vi "NEW数据采集传输系统.vi"() -> ()   [LabVIEW 2016, in "数据传输系统-05.lvlib"]
uses:
  <vilib>/Utility/miscctls.llb/LVPointTypeDef.ctl
  <vilib>/Utility/error.llb/whitespace.ctl
  <vilib>/picture/picture.llb/imagedata.ctl
  <vilib>/Utility/config.llb/NI_LVConfig.lvlib
  update/update.lvlib
panel:
  out "剖面数据补发":bool
  out "日志信息补发":bool
  out "数据补发":bool
  in  "自动更新":bool
  in  "数据补传":bool caption="确定"
  out "数据库打开失败次数":dbl
  out "与工控通信指示灯":bool
  in  "判断数据反馈":enum16{"非严格判断", "严格判断", "不判断"}(ring)
  in  "暂停上传":bool
  in  "配置表":bool caption="确定"
  in  "updateconfiguration":T1={"主机"="27.154.58.30", "用户"="update", "密码"="std23506", "远程路径"="数据传输系统\\平台数据传输系统.exe", "下载文件名"="平台数据传输系统.exe", "软件版本"=""}
  out "标题显示":string
  in  "更新":bool
  in  "系统编码选择框":string(combo)="地表水质量监测"
  in  "数据发送通道":enum16{"TCP", "VISA"}(ring)
  in  "baud rate":u32=9600 caption="波特率"
  in  "VISA resource name":refnum<visa-resource-name> caption="VISA资源名称"
  in  "实时数据发送时间间隔/min":i32=1
  in  "数据组合发送":bool
  in  "2011发送":bool
  in  "数据发送协议":enum16{"2005-212协议", "2017-212协议"}(ring)=enum."2017-212协议"
  in  "重发时间":T2(ring)
  in  "重发日期":T3(ring)
  in  "开机启动":bool
  in  "每周自动重发":bool=TRUE
  in  "确定":bool
  in  "返回":bool
  in  "PW":string
  in  "MN":string
  in  "PORT":string
  in  "IP":string
  in  "站点设备":string
  in  "站点名称":string
  out "设置超时时间/min":i32=1
  out "状态信息":T4={"1st Error to Convert "=63, "步骤 "=enum."发送数据", "元素"="实时数据", "TCP服务端掉线计数"=0, "TCP掉线时间节点"="2019/05/08 15:24:17"} {"1st Error to Convert" items=["无错误", "参数错误", "内存已满", "超出区域", "文件结束", "文件已打开", "一般文件IO错误", "未找到文件", "文件权限错误", "磁盘已满", "路径副本", "打开过多文件", "未启用", "未找到资源文件", "无法添加资源", "未找到资源", "未找到图像", "图像内存错误", "画笔不存在", "配置错误类型", "配置未找到解析段", "配置解析错误", "配置内存错误", "错误外部代码格式", "错误外部代码偏移量", "外部代码不存在", "空窗口", "销毁窗口错误", "空菜单", "打印已中止", "错误打印记录", "打印驱动程序错误", "打印时窗口错误", "打印时内存错误", "打印对话框错误", "一般打印错误", "无效设备引用句柄", "设备未找到", "设备参数错误", "设备单位错误", "无法打开设备", "设备调用已中止", "一般错误", "用户已取消", "对象ID过低", "对象ID过高", "对象不在堆中", "未知的堆", "错误DefProc ID", "DefProc不在表格中", "范围外信息", "空方法", "未知信息", "不支持管理器调用", "错误地址", "连接过程中", "连接超时", "连接过程中", "不支持网络属性", "网络错误", "正在使用的地址", "系统缺少内存", "连接已中止", "连接已拒绝", "连接未建立", "连接已建立", "连接已关闭", "初始化错误（交互应用程序管理器）", "错误事件发生", "等待无约束事件发生处理程序", "事件发生队列溢出", "错误路径", "未发出信号量", "未识别类型（交互应用程序管理器）"]}
  out "数据接收超时指示灯":bool
  out "空闲时间/s":string
  out "系统时间":string
  out "实时小时数据上传":bool
  out "系统状态改变":bool
  out "软件版本":string
  out "掉线指示":bool
  out "核查数据上传":bool
  out "配置信息":T5
  in  "参数配置":bool
  out "反控数据发送":bool
  out "读取报文显示":string
  out "发送报文显示":string
  out "心跳包":bool
  out "通信状态":bool
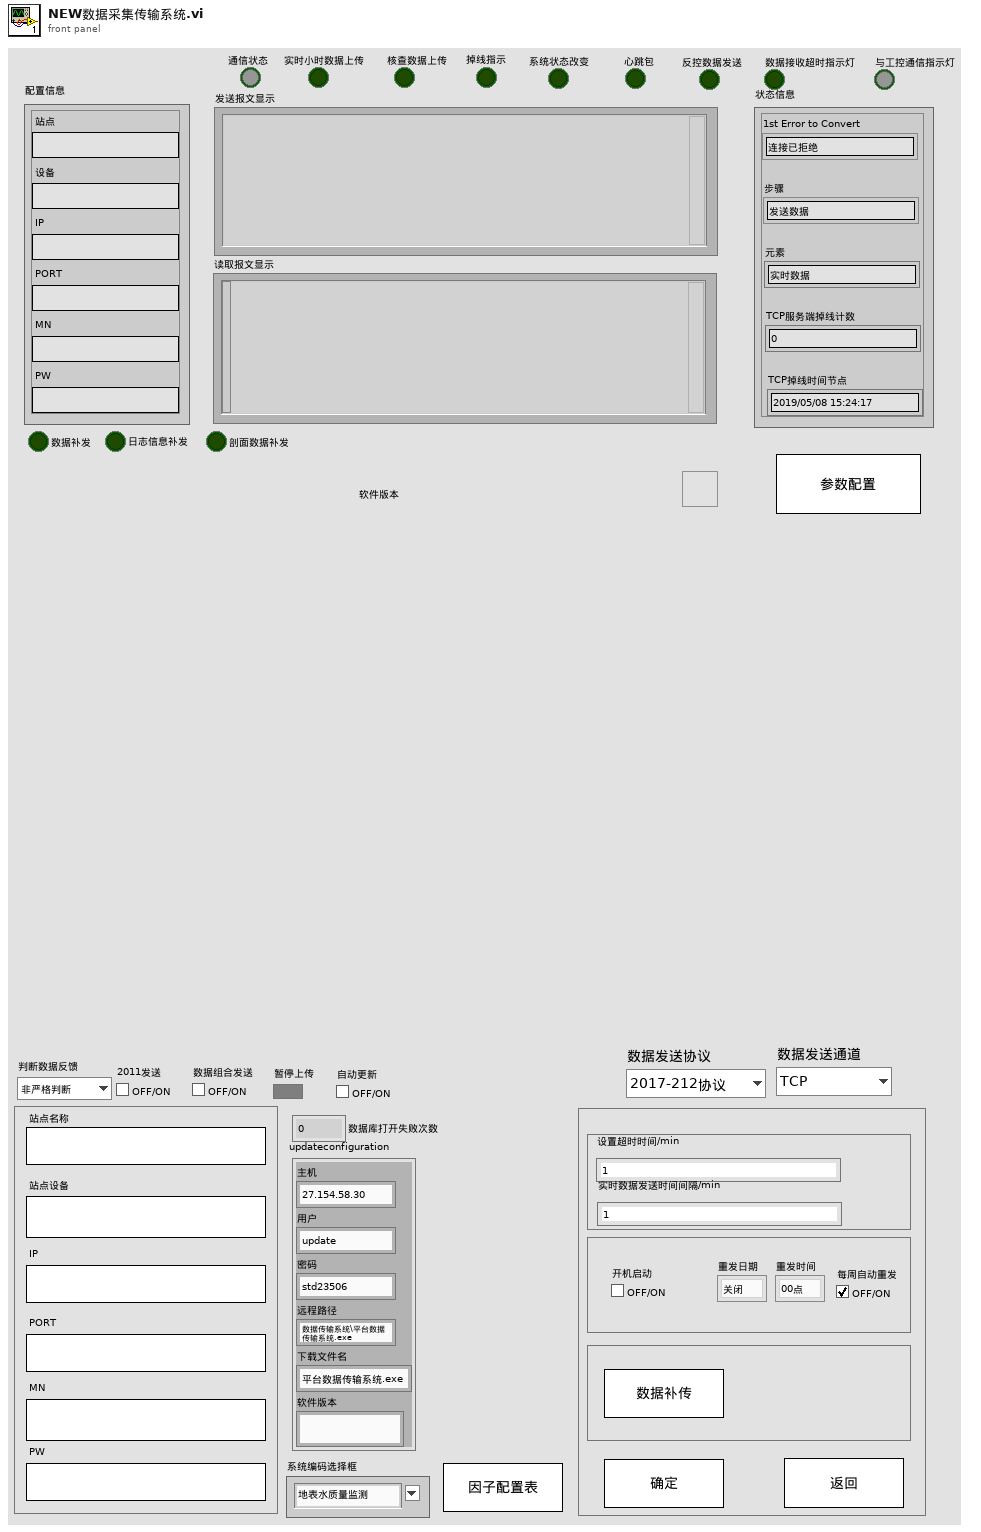
[diagram p1: front panel]
types:
  T1 = cluster{"主机":string, "用户":string, "密码":string, "远程路径":string, "下载文件名":string, "软件版本":string}
  T2 = enum16{"00点", "01点", "02点", "03点", "04点", "05点", "06点", "07点", "08点", "09点", "10点", "11点", "12点", "13点", "14点", "15点", "16点", "17点", "18点", "19点", "20点", "21点", "22点", "23点"}
  T3 = enum16{"关闭", "星期日", "星期一", "星期二", "星期三", "星期四", "星期五", "星期六"}
  T4 = cluster{"1st Error to Convert ":i32, "步骤 ":enum16{"打开连接", "发送数据", "读取数据", "数据处理", "关闭连接"}, "元素":string, "TCP服务端掉线计数":i32, "TCP掉线时间节点":string}
  T5 = cluster{"站点":string, "设备":string, "IP":string, "PORT":string, "MN":string, "PW":string}
  T6 = typedef "imagedata.ctl" = cluster{"image type":i32, "image depth":i32, "image":u8[], "mask":u8[], "colors":u32[], "Rectangle":cluster{"left":i16, "top":i16, "right":i16, "bottom":i16}}
  T7 = typedef "LVPointTypeDef.ctl" = cluster{"Horizontal":i16, "Vertical":i16}
  T8 = cluster{"setini":string, "sysini":string, "hechaini":string, "actualwrite":string, "actualread":string, "datasent":string, "反控命令信息队列":string, "反控与仪器交互":string}
  T9 = cluster{"配置表格[0]":string, "配置表格[1]":string, "配置表格[2]":string, "配置表格[3]":string, "配置表格[4]":string, "配置表格[5]":string, "配置表格[6]":string, "配置表格[7]":string, "配置表格[8]":string, "配置表格[9]":string, "配置表格[10]":string, "配置表格[11]":string, "配置表格[12]":string, "配置表格[13]":string, "配置表格[14]":string, "配置表格[15]":string, "配置表格[16]":string, "配置表格[17]":string, "配置表格[18]":string, "配置表格[19]":string, "配置表格[20]":string, "配置表格[21]":string, "配置表格[22]":string, "配置表格[23]":string, "配置表格[24]":string, "配置表格[25]":string, "配置表格[26]":string, "配置表格[27]":string, "配置表格[28]":string, "配置表格[29]":string, "配置表格[30]":string, "配置表格[31]":string, "配置表格[32]":string, "配置表格[33]":string, "配置表格[34]":string}
  T10 = cluster{"[0]":dbl, "[1]":dbl, "[2]":dbl, "[3]":dbl, "[4]":dbl, "[5]":dbl, "[6]":dbl, "[7]":dbl, "[8]":dbl, "[9]":dbl, "[10]":dbl, "[11]":dbl, "[12]":dbl, "[13]":dbl, "[14]":dbl, "[15]":dbl, "[16]":dbl, "[17]":dbl, "[18]":dbl, "[19]":dbl, "[20]":dbl, "[21]":dbl, "[22]":dbl, "[23]":dbl, "[24]":dbl, "[25]":dbl, "[26]":dbl, "[27]":dbl, "[28]":dbl, "[29]":dbl, "[30]":dbl, "[31]":dbl, "[32]":dbl, "[33]":dbl, "[34]":dbl}
  T11 = cluster{"时间标识":timestamp, "设备":string, "日志信息":string, "流程参数":string}
  T12 = cluster{"host":string, "port":u16, "user":string, "password":string, "远端地址":string}
  T13 = typedef "NI_LVConfig.lvlib/Config Data RefNum.ctl" = refnum<k1>
  T14 = cluster{"[0]":string, "[1]":string, "[2]":string, "[3]":string, "[4]":string, "[5]":string, "[6]":string}
  T15 = cluster{"[0]":string, "[1]":string, "[2]":string, "[3]":string, "[4]":string, "[5]":string, "[6]":string, "[7]":string, "[8]":string}
  T16 = cluster{"[0]":string, "[1]":string, "[2]":string, "[3]":string, "[4]":string, "[5]":string}
  T17 = cluster{"[0]":string, "[1]":string, "[2]":string, "[3]":string, "[4]":string, "[5]":string, "[6]":string, "[7]":string, "[8]":string, "[9]":string, "[10]":string, "[11]":string, "[12]":string, "[13]":string, "[14]":string, "[15]":string}
  T18 = cluster{"[0]":string, "[1]":string, "[2]":string, "[3]":string, "[4]":string, "[5]":string, "[6]":string, "[7]":string, "[8]":string, "[9]":string, "[10]":string, "[11]":string, "[12]":string, "[13]":string}
  T19 = cluster{"[0]":string, "[1]":string, "[2]":string, "[3]":string, "[4]":string, "[5]":string, "[6]":string, "[7]":string, "[8]":string, "[9]":string, "[10]":string, "[11]":string, "[12]":string, "[13]":string, "[14]":string, "[15]":string, "[16]":string, "[17]":string, "[18]":string, "[19]":string, "[20]":string, "[21]":string, "[22]":string, "[23]":string, "[24]":string, "[25]":string, "[26]":string, "[27]":string, "[28]":string, "[29]":string, "[30]":string, "[31]":string, "[32]":string, "[33]":string, "[34]":string}
  T20 = typedef "whitespace.ctl" = u16
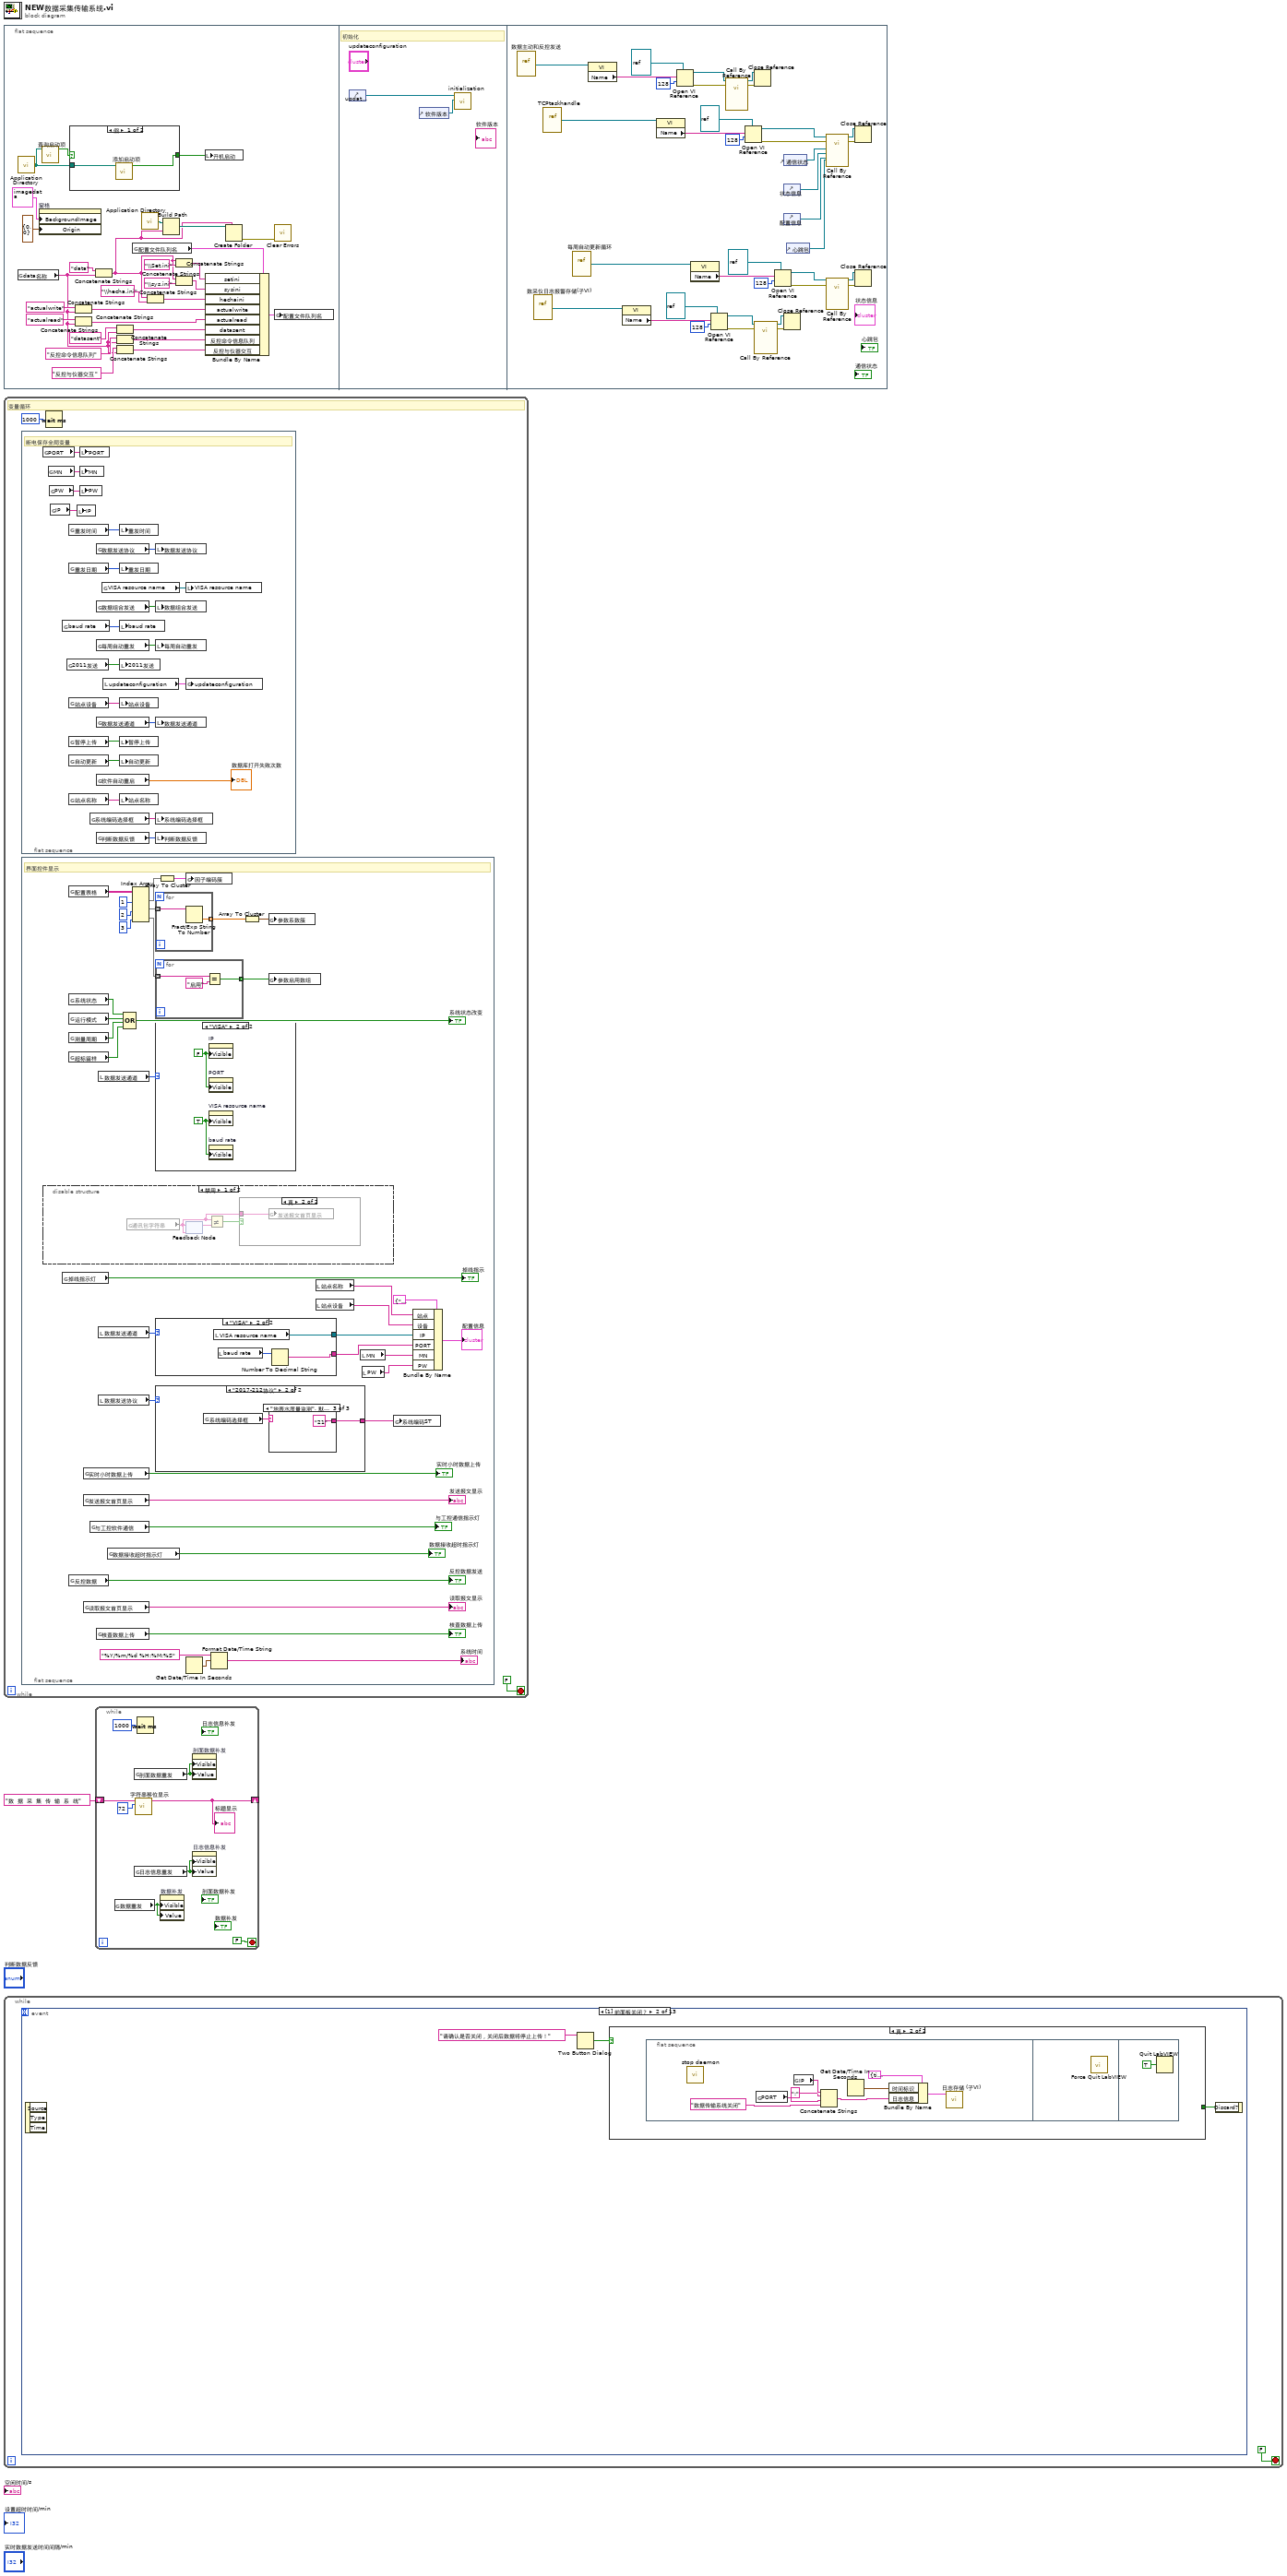
[diagram p0: block diagram]
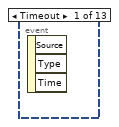
[diagram p2: hidden frame]
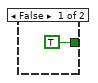
[diagram p3: hidden frame]
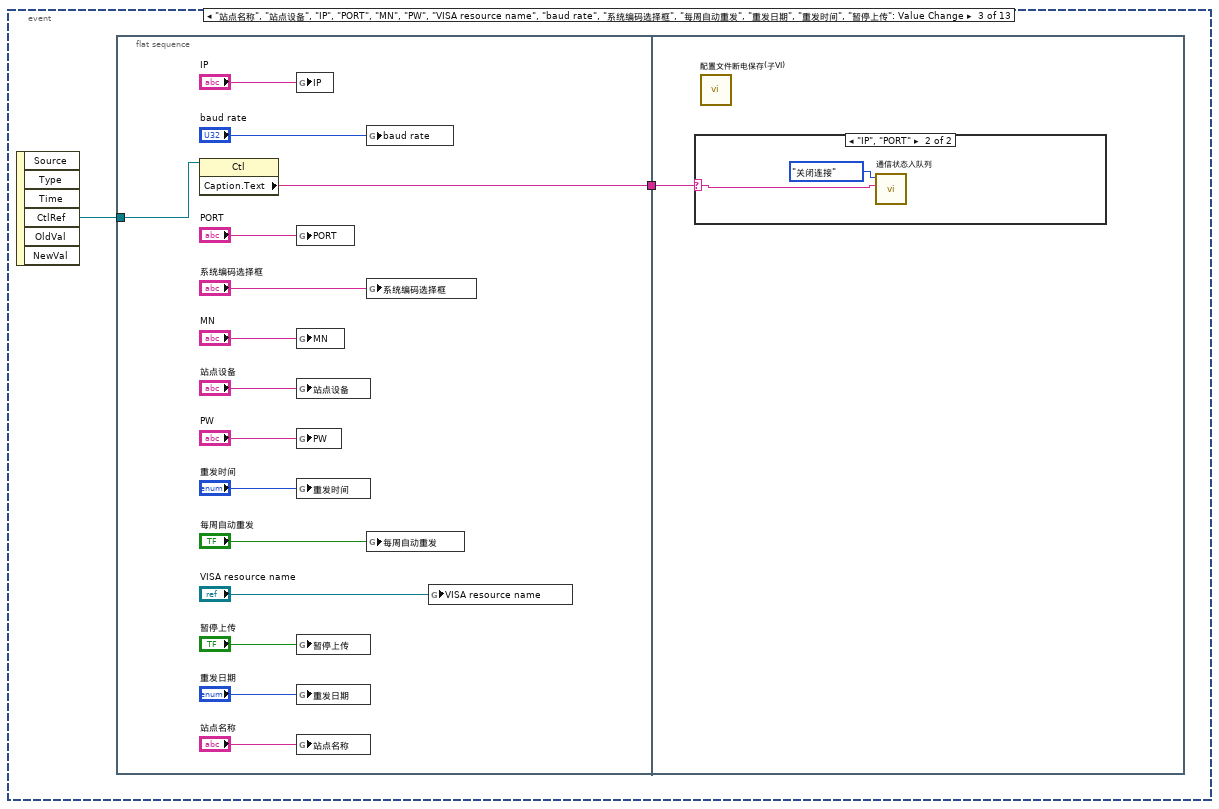
[diagram p4: hidden frame]
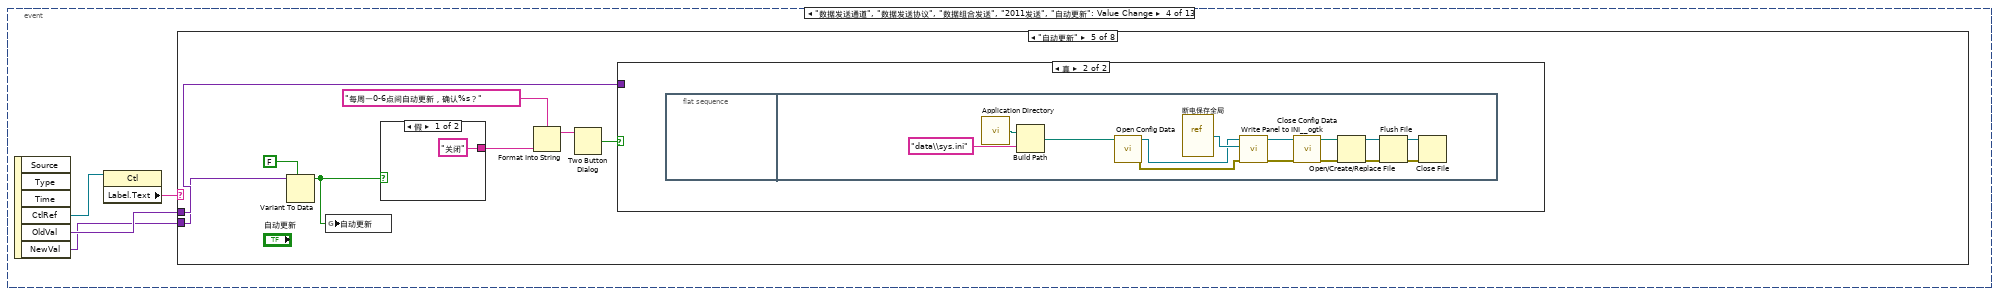
[diagram p6: hidden frame]
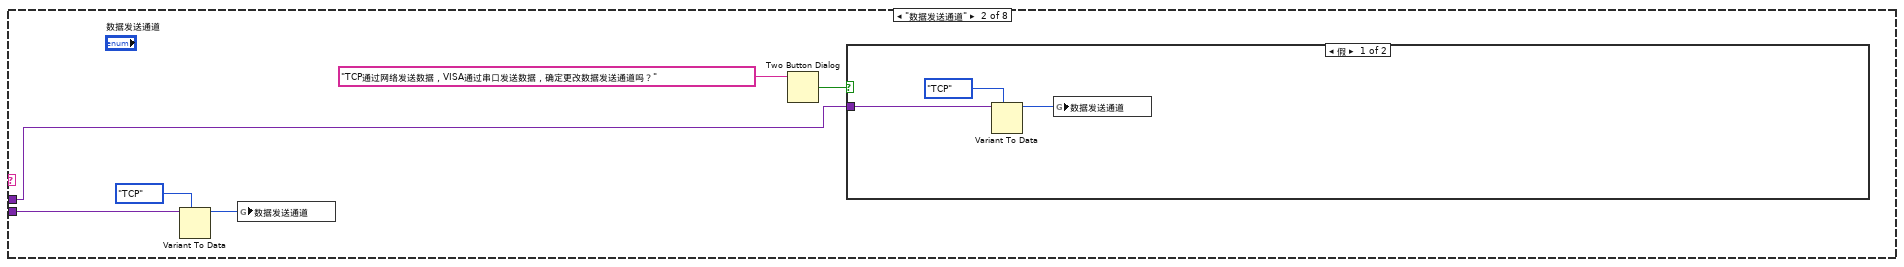
[diagram p8: hidden frame]
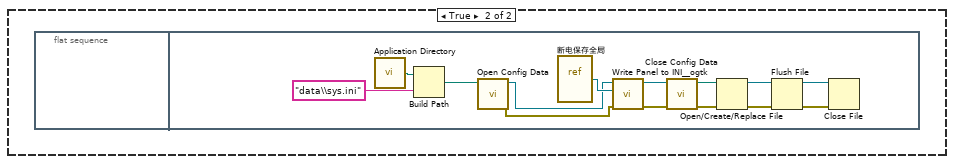
[diagram p9: hidden frame]
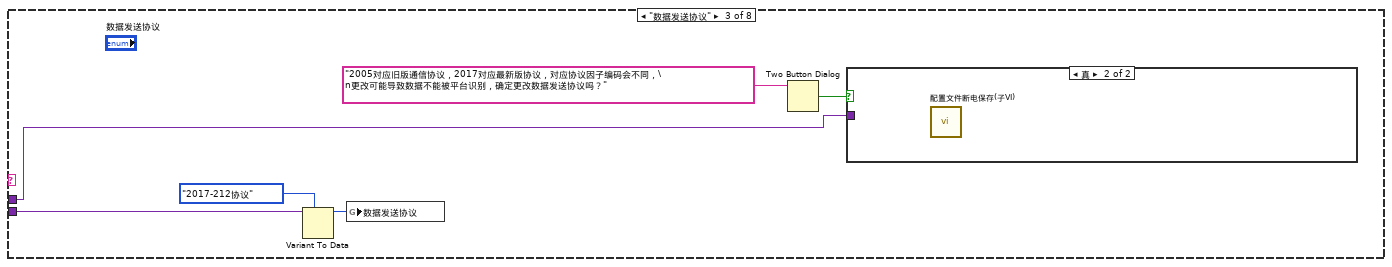
[diagram p10: hidden frame]
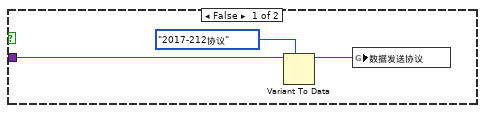
[diagram p11: hidden frame]
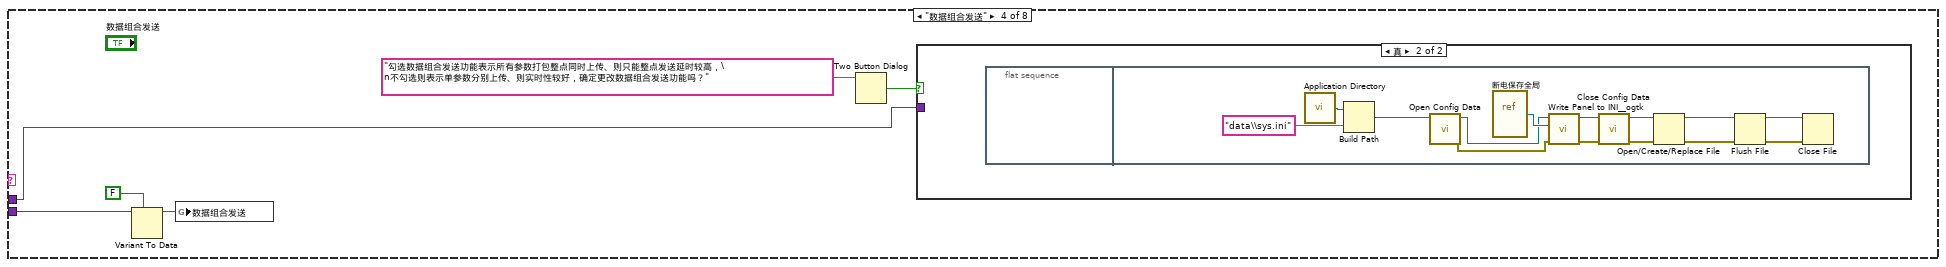
[diagram p12: hidden frame]
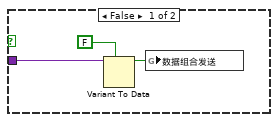
[diagram p13: hidden frame]
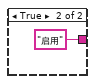
[diagram p14: hidden frame]
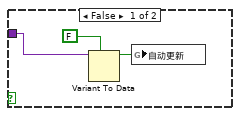
[diagram p15: hidden frame]
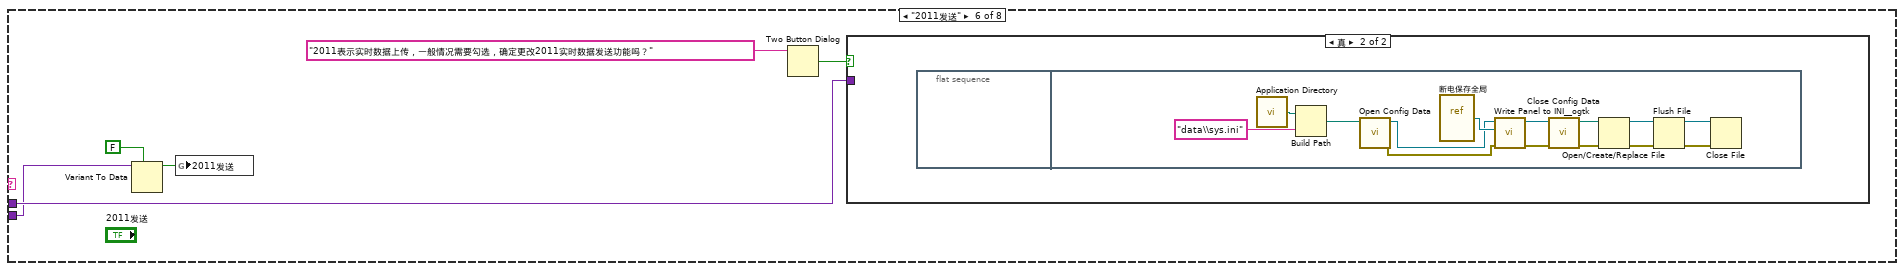
[diagram p16: hidden frame]
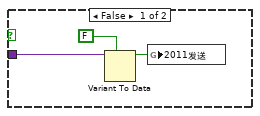
[diagram p17: hidden frame]
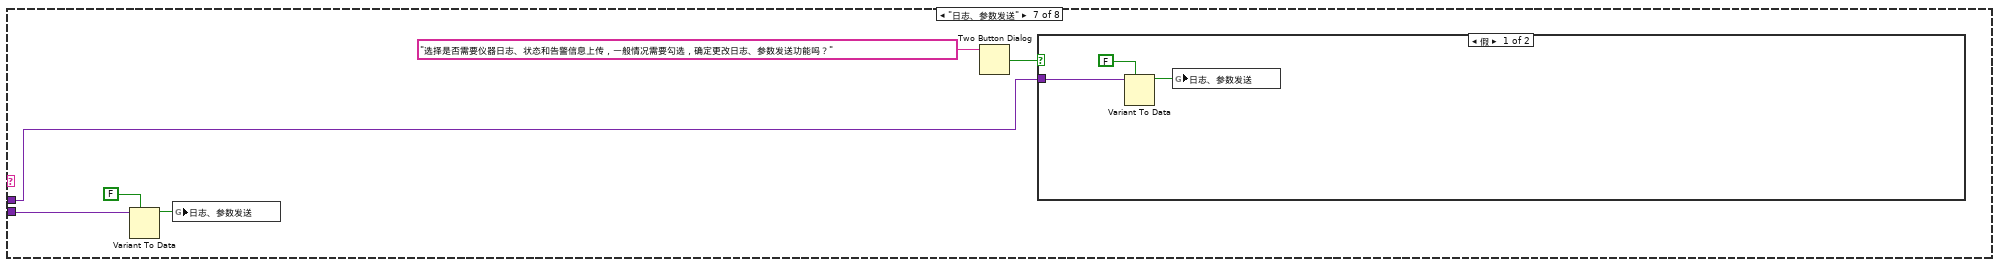
[diagram p18: hidden frame]
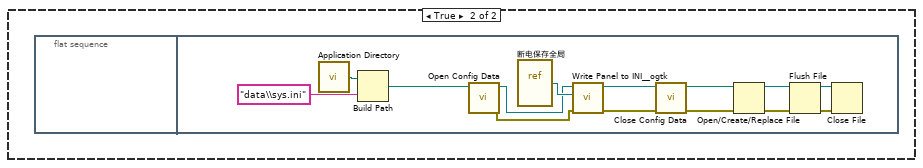
[diagram p19: hidden frame]
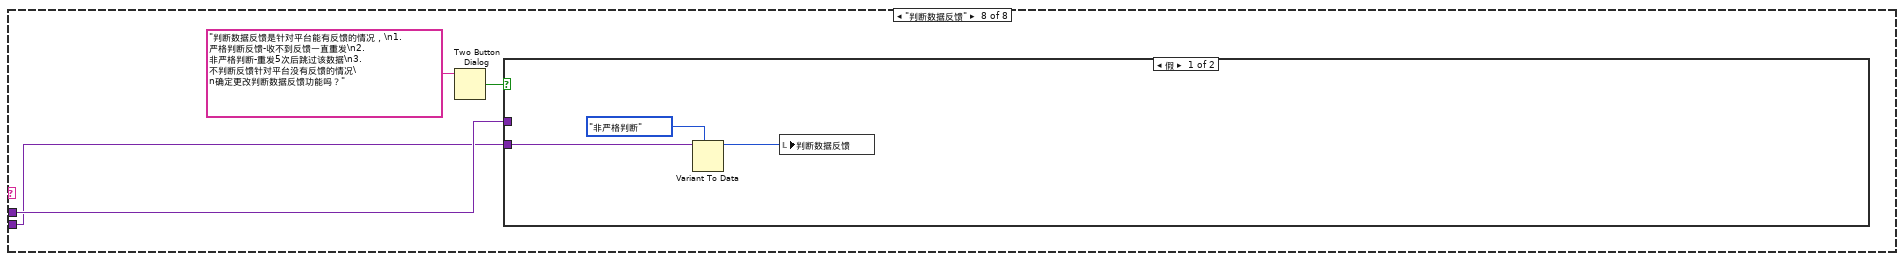
[diagram p20: hidden frame]
diagram:
  n1 = flat-sequence {
    frame #0 {
      n2 = global read "断电保存全局.vi" "data名称"() -> (w2:string)
      n3 = call <vilib>:"Application Directory.vi"() -> ("Application Directory"=w6:path)
      n4 = property on="窗格" class="Pane"("BackgroundImage"=T6 {"image type"=0, "image depth"=24, "image"=array[12288000 elements], "mask"=[], "colors"=[], "Rectangle"={"left"=0, "top"=0, "right"=2560, "bottom"=1600}} ("image data"), "Origin"=T7 {"Horizontal"=0, "Vertical"=0} ("原点")) -> ()  [unwired: 2 in, 2 out]
      n5 = call "查询启动项.vi"("启动文件路径"=w6) -> ("包含启动项"=w5:bool)  [unwired: 9 in, 1 out]
      n6 = case shown="假" w5 {
        selector: w5 -> [_ w33]
        tunnel: w6 -> [w32 _]
        tunnel: [w31 w33] -> w4
        frame False {
          n7 = call "添加启动项.vi"("启动文件路径"=w32) -> ("添加成功标记"=w31:bool)  [unwired: 9 in, 1 out]
        }
        frame True {
        }
      }
      n8 = Concatenate Strings("actualwrite" ("名称（未命名）"), w2) -> (w18:string)
      n9 = Concatenate Strings("actualread" ("名称（未命名）"), w2) -> (w16:string)
      n10 = Concatenate Strings("data" ("对话框窗口（创建文件夹）"), w2) -> (w23:string)
      n11 = Concatenate Strings("datasent" ("名称（未命名）"), w2) -> (w14:string)
      n12 = Concatenate Strings("反控命令信息队列" ("名称（未命名）"), w2) -> (w8:string)
      n13 = Concatenate Strings("反控与仪器交互" ("名称（未命名）"), w2) -> (w9:string)
      n14 = global read "断电保存全局.vi" "配置文件队列名"() -> (w13:T8)
      n15 = call <vilib>:"Application Directory.vi"() -> ("Application Directory"=w29:path)
      n16 = Concatenate Strings(w23, "\\hecha.ini" ("名称或相对路径")) -> (w21:string)
      n17 = Build Path(base path=w29, name or relative path=w23) -> (appended path=w28:path)
      n18 = Concatenate Strings(w23, "\\Set.ini" ("名称或相对路径")) -> (w25:string)
      n19 = Concatenate Strings(w23, "\\sys.ini" ("名称或相对路径")) -> (w22:string)
      n20 = local write "开机启动"(w4) -> ()
      n21 = Bundle By Name(cluster=w13, "setini"=w25, "sysini"=w22, "hechaini"=w21, "actualwrite"=w18, "actualread"=w16, "datasent"=w14, "反控命令信息队列"=w8, "反控与仪器交互"=w9) -> (w12:T8)
      n22 = Create Folder(prompt (Create Folder)=w23, path (use dialog)=w28) -> (error out=w27:errorcluster)  [unwired: 1 in, 2 out]
      n23 = call <vilib>:"Clear Errors.vi"("error in (no error)"=w27) -> ()  [unwired: 5 in, 2 out]
      n24 = global write "断电保存全局.vi" "配置文件队列名"(w12) -> ()
    }
    frame #1 {
      # "初始化"
      n25 = control-ref of="updateconfiguration"() -> (w35:refnum<vi>)
      n26 = control-ref of="软件版本"() -> (w34:refnum<vi>)
      n27 = call "initialization.vi"("软件版本"=w34, "updateconfiguration"=w35) -> ()  [unwired: 9 in]
    }
    frame #2 {
      n28 = vi-ref "数据主动和反控发送.vi"() -> (w63:refnum<vi>)
      n29 = vi-ref "数采仪日志报警存储(子VI).vi"() -> (w64:refnum<vi>)
      n30 = vi-ref "TCPtaskhandle.vi"() -> (w40:refnum<vi>)
      n31 = vi-ref "每周自动更新循环.vi"() -> (w55:refnum<vi>)
      n32 = property class="VI"(reference=w63) -> ("Name"=w62:string)  [unwired: 1 in, 2 out]
      n33 = property class="VI"(reference=w64) -> ("Name"=w71:string)  [unwired: 1 in, 2 out]
      n34 = property class="VI"(reference=w40) -> ("Name"=w47:string)  [unwired: 1 in, 2 out]
      n35 = Open VI Reference(type specifier VI Refnum (for type only)=refnum<vi> refnum, vi path=w62, options=128 ("选项")) -> (vi reference=w60:refnum<vi>, error out=w58:errorcluster)  [unwired: 3 in]
      n36 = property class="VI"(reference=w55) -> ("Name"=w48:string)  [unwired: 1 in, 2 out]
      n37 = Open VI Reference(type specifier VI Refnum (for type only)=refnum<vi> refnum, vi path=w71, options=128 ("选项")) -> (vi reference=w69:refnum<vi>, error out=w67:errorcluster)  [unwired: 3 in]
      n38 = call-by-ref "?"(reference=w60, error in=w58) -> (reference out=w56:refnum<vi>, error out=w57:errorcluster)  [unwired: 12 in]
      n39 = Open VI Reference(type specifier VI Refnum (for type only)=refnum<vi> refnum, vi path=w47, options=128 ("选项")) -> (vi reference=w45:refnum<vi>, error out=w43:errorcluster)  [unwired: 3 in]
      n40 = Close Reference(reference=w56, error in (no error)=w57) -> ()  [unwired: 1 out]
      n41 = call-by-ref "?"(reference=w69, error in=w67) -> (reference out=w65:refnum<vi>, error out=w66:errorcluster)  [unwired: 12 in]
      n42 = Open VI Reference(type specifier VI Refnum (for type only)=refnum<vi> refnum, vi path=w48, options=128 ("选项")) -> (vi reference=w50:refnum<vi>, error out=w52:errorcluster)  [unwired: 3 in]
      n43 = control-ref of="通信状态"() -> (w39:refnum<vi>)
      n44 = control-ref of="状态信息"() -> (w38:refnum<vi>)
      n45 = control-ref of="配置信息"() -> (w37:refnum<vi>)
      n46 = Close Reference(reference=w65, error in (no error)=w66) -> ()  [unwired: 1 out]
      n47 = control-ref of="心跳包"() -> (w36:refnum<vi>)
      n48 = call-by-ref "?"(reference=w45, error in=w43, "心跳包"=w36, "配置信息"=w37, "状态信息"=w38, "通信状态"=w39) -> (reference out=w41:refnum<vi>, error out=w42:errorcluster)  [unwired: 8 in]
      n49 = call-by-ref "?"(reference=w50, error in=w52) -> (reference out=w54:refnum<vi>, error out=w53:errorcluster)  [unwired: 12 in]
      n50 = Close Reference(reference=w41, error in (no error)=w42) -> ()  [unwired: 1 out]
      n51 = Close Reference(reference=w54, error in (no error)=w53) -> ()  [unwired: 1 out]
    }
  }
  n52 = while {
    stop <- FALSE stop-if-true
    # "变量循环"
    n53 = flat-sequence {
      frame #0 {
        # "断电保存全局变量"
        n54 = global read "断电保存全局.vi" "PORT"() -> (w158:string)
        n55 = global read "断电保存全局.vi" "MN"() -> (w157:string)
        n56 = global read "断电保存全局.vi" "PW"() -> (w156:string)
        n57 = global read "断电保存全局.vi" "IP"() -> (w159:string)
        n58 = global read "断电保存全局.vi" "baud rate"() -> (w154:u32)
        n59 = global read "断电保存全局.vi" "2011发送"() -> (w150:bool)
        n60 = global read "断电保存全局.vi" "重发时间"() -> (w145:T2)
        n61 = global read "断电保存全局.vi" "重发日期"() -> (w152:T3)
        n62 = global read "断电保存全局.vi" "站点设备"() -> (w160:string)
        n63 = global read "断电保存全局.vi" "暂停上传"() -> (w143:bool)
        n64 = global read "断电保存全局.vi" "自动更新"() -> (w141:bool)
        n65 = global read "断电保存全局.vi" "站点名称"() -> (w161:string)
        n66 = local write "IP"(w159) -> ()
        n67 = local write "PORT"(w158) -> ()
        n68 = local write "MN"(w157) -> ()
        n69 = local write "PW"(w156) -> ()
        n70 = global read "断电保存全局.vi" "系统编码选择框"() -> (w146:string)
        n71 = global read "断电保存全局.vi" "数据发送协议"() -> (w148:enum16{"2005-212协议", "2017-212协议"})
        n72 = global read "断电保存全局.vi" "数据组合发送"() -> (w149:bool)
        n73 = global read "断电保存全局.vi" "每周自动重发"() -> (w153:bool)
        n74 = global read "断电保存全局.vi" "数据发送通道"() -> (w147:enum16{"TCP", "VISA"})
        n75 = global read "全局1.vi" "软件自动重启"() -> (→"数据库打开失败次数":dbl)
        n76 = global read "断电保存全局.vi" "判断数据反馈"() -> (w151:enum16{"非严格判断", "严格判断", "不判断"})
        n77 = global read "断电保存全局.vi" "VISA resource name"() -> (w155:refnum<visa-resource-name>)
        n78 = local read "updateconfiguration"() -> (w144:T1)
        n79 = local write "重发时间"(w145) -> ()
        n80 = local write "重发日期"(w152) -> ()
        n81 = local write "baud rate"(w154) -> ()
        n82 = local write "2011发送"(w150) -> ()
        n83 = local write "站点设备"(w160) -> ()
        n84 = local write "暂停上传"(w143) -> ()
        n85 = local write "自动更新"(w141) -> ()
        n86 = local write "站点名称"(w161) -> ()
        n87 = local write "数据发送协议"(w148) -> ()
        n88 = local write "数据组合发送"(w149) -> ()
        n89 = local write "每周自动重发"(w153) -> ()
        n90 = local write "数据发送通道"(w147) -> ()
        n91 = local write "系统编码选择框"(w146) -> ()
        n92 = local write "判断数据反馈"(w151) -> ()
        n93 = local write "VISA resource name"(w155) -> ()
        n94 = global write "更新全局变量.vi" "updateconfiguration"(w144) -> ()
      }
    }
    n95 = flat-sequence {
      frame #0 {
        # "界面控件显示"
        n96 = disable-structure shown="禁用" {
          frame Disabled {
            n97 = global read "全局1.vi" "通讯包字符串"() -> (w114:string)
            n98 = feedback #1(w114) -> (w115:string)
            n99 = feedback-in #1(w114) -> ()
            n100 = Not Equal?(x=w114, y=w115) -> (x != y?=w113:bool)
            n101 = case shown="真" w113 {
              tunnel: w114 -> [_ w116]
              frame False {
              }
              frame True {
                n102 = global write "全局1.vi" "发送报文首页显示"(w116) -> ()
              }
            }
          }
          frame Enabled {
          }
        }
        n103 = global read "全局 数据发送重叠.vi" "掉线指示灯"() -> (→"掉线指示":bool)
        n104 = global read "断电保存全局.vi" "配置表格"() -> (w84:string[][])
        n105 = global read "全局1.vi" "系统状态"() -> (w86:bool)
        n106 = global read "全局1.vi" "运行模式"() -> (w87:bool)
        n107 = global read "全局1.vi" "测量周期"() -> (w88:bool)
        n108 = global read "全局1.vi" "超标留样"() -> (w89:bool)
        n109 = global read "全局1.vi" "反控数据"() -> (→"反控数据发送":bool)
        n110 = global read "全局1.vi" "实时小时数据上传"() -> (→"实时小时数据上传":bool)
        n111 = global read "全局1.vi" "发送报文首页显示"() -> (→"发送报文显示":string)
        n112 = global read "全局1.vi" "读取报文首页显示"() -> (→"读取报文显示":string)
        n113 = global read "全局1.vi" "与工控软件通信"() -> (→"与工控通信指示灯":bool)
        n114 = global read "全局1.vi" "核查数据上传"() -> (→"核查数据上传":bool)
        n115 = local read "数据发送通道"() -> (w94:enum16{"TCP", "VISA"})
        n116 = local read "数据发送通道"() -> (w112:enum16{"TCP", "VISA"})
        n117 = local read "数据发送协议"() -> (w101:enum16{"2005-212协议", "2017-212协议"})
        n118 = global read "全局 数据发送重叠.vi" "数据接收超时指示灯"() -> (→"数据接收超时指示灯":bool)
        n119 = Compound Arithmetic op=OR ("复合运算")(w86, w87, w88, w89) -> (→"系统状态改变":bool)
        n120 = Index Array(array=w84, index (col) #1=1 ("禁用的索引 (列)"), index (col) #2=2 ("索引 (列)"), index (col) #3=3 ("索引 (列)")) -> (element #1=w82:string[], element #2=w76:string[], element #3=w78:string[])  [unwired: 3 in]
        n121 = for {
          tunnel: w76 -> [w118] mode=indexing
          tunnel: [w117] -> w75 mode=indexing
          n122 = Fract/Exp String To Number(string=w118) -> (number=w117:dbl)  [unwired: 3 in, 1 out]
        }
        n123 = for {
          tunnel: w78 -> [w121] mode=indexing
          tunnel: [w119] -> w77 mode=indexing
          n124 = Equal?(x=w121, y="启用") -> (x = y?=w119:bool)
        }
        n125 = case shown="\"VISA\"" w94 {
          frame "TCP", Default {
            w122 = TRUE ("可见")
            w123 = FALSE ("可见")
            n126 = property on="IP" class="Str"("Visible"=w122) -> ()  [unwired: 2 in, 2 out]
            n127 = property on="PORT" class="Str"("Visible"=w122) -> ()  [unwired: 2 in, 2 out]
            n128 = property on="VISA resource name" class="VISAName"("Visible"=w123) -> ()  [unwired: 2 in, 2 out]
            n129 = property on="baud rate" class="DigNum (严格)"("Visible"=w123) -> ()  [unwired: 2 in, 2 out]
          }
          frame "VISA" {
            w124 = FALSE ("可见")
            w125 = TRUE ("可见")
            n130 = property on="IP" class="Str"("Visible"=w124) -> ()  [unwired: 2 in, 2 out]
            n131 = property on="PORT" class="Str"("Visible"=w124) -> ()  [unwired: 2 in, 2 out]
            n132 = property on="VISA resource name" class="VISAName"("Visible"=w125) -> ()  [unwired: 2 in, 2 out]
            n133 = property on="baud rate" class="DigNum (严格)"("Visible"=w125) -> ()  [unwired: 2 in, 2 out]
          }
        }
        n134 = case shown="\"VISA\"" w112 {
          tunnel: [w137 w140] -> w109
          tunnel: [w136 w138] -> w106
          frame "TCP", Default {
            n135 = local read "PORT"() -> (w136:string)
            n136 = local read "IP"() -> (w137:string)
          }
          frame "VISA" {
            n137 = local read "VISA resource name"() -> (w140:refnum<visa-resource-name>)
            n138 = local read "baud rate"() -> (w139:u32)
            n139 = Number To Decimal String(number=w139) -> (decimal integer string=w138:string)  [unwired: 1 in]
          }
        }
        n140 = case shown="\"2017-212协议\"" w101 {
          tunnel: [w126 w131] -> w100
          frame "2005-212协议", Default {
            n141 = global read "断电保存全局.vi" "系统编码选择框"() -> (w127:string)
            n142 = case shown="\"地表水体污染源\"" w127 {
              tunnel: ["52" ("设备编码MN") "32" ("设备编码MN") "21" ("设备编码MN")] -> w126
              frame "污水排放过程监测" {
              }
              frame "地表水体污染源" {
              }
              frame "地表水质量监测", Default {
              }
            }
          }
          frame "2017-212协议" {
            n143 = global read "断电保存全局.vi" "系统编码选择框"() -> (w132:string)
            n144 = case shown="\"地表水质量监测\", 默认" w132 {
              tunnel: ["52" ("设备编码MN") "32" ("设备编码MN") "21" ("设备编码MN")] -> w131
              frame "污水排放过程监测" {
              }
              frame "地表水体污染源" {
              }
              frame "地表水质量监测", Default {
              }
            }
          }
        }
        n145 = Array To Cluster(array=w82) -> (cluster=w85:T9)
        n146 = global write "断电保存全局.vi" "因子编码簇"(w85) -> ()
        n147 = Get Date/Time In Seconds() -> (seconds since 1Jan1904=w102:timestamp)
        n148 = Format Date/Time String(time format string (%c)="%Y/%m/%d %H:%M:%S" ("时间格式字符串(%c)"), seconds (now)=w102) -> (date/time string=→"系统时间":string)  [unwired: 1 in]
        n149 = Array To Cluster(array=w75) -> (cluster=w79:T10)
        n150 = global write "断电保存全局.vi" "参数系数簇"(w79) -> ()
        n151 = global write "断电保存全局.vi" "参数启用数组"(w77) -> ()
        n152 = local read "站点名称"() -> (w108:string)
        n153 = local read "站点设备"() -> (w107:string)
        n154 = local read "MN"() -> (w105:string)
        n155 = local read "PW"() -> (w104:string)
        n156 = global write "全局1.vi" "系统编码ST"(w100) -> ()
        n157 = Bundle By Name(cluster=T5 {"站点"="", "设备"="", "IP"="", "PORT"="", "MN"="", "PW"=""} ("配置信息"), "站点"=w108, "设备"=w107, "IP"=w109, "PORT"=w106, "MN"=w105, "PW"=w104) -> (→"配置信息":T5)
      }
    }
    n158 = Wait (ms)(milliseconds to wait=u32 1000 ("等待时间（毫秒）")) -> ()  [unwired: 1 out]
  }
  n159 = while {
    stop <- FALSE stop-if-true
    n160 = event shown="[1] 前面板关闭？" {
      selector: _ -> [_ _ _ _ _ _ _ _ _ _ _ _ _]
      dyn-events: _ -> [_ _ _ _ _ _ _ _ _ _ _ _ _]
      timeout: _ -> [_ _ _ _ _ _ _ _ _ _ _ _ _]
      event Timeout {
        n161 = event-data() -> ()  [unwired: 1 in, 3 out]
      }
      event Panel Close? {
        n162 = event-data() -> ()  [unwired: 1 in, 3 out]
        n163 = Two Button Dialog(message="请确认是否关闭，关闭后数据将停止上传！" ("消息")) -> (T button?=w164:bool)  [unwired: 2 in]
        n164 = case shown="真" w164 {
          tunnel: [TRUE _] -> w163
          frame False {
          }
          frame True {
            n165 = flat-sequence {
              frame #0 {
                n166 = call "stop daemon.vi"() -> ()  [unwired: 11 in, 1 out]
                n167 = global read "断电保存全局.vi" "PORT"() -> (w170:string)
                n168 = global read "断电保存全局.vi" "IP"() -> (w172:string)
                n169 = Concatenate Strings(w172, ":", w170, "数据传输系统关闭" ("日志信息")) -> (w168:string)
                n170 = Get Date/Time In Seconds() -> (seconds since 1Jan1904=w174:timestamp)
                n171 = Bundle By Name(cluster=T11 {"时间标识"=timestamp(0 s since 1904-01-01), "设备"="数采仪", "日志信息"="", "流程参数"=""} ("data in"), "时间标识"=w174, "日志信息"=w168) -> (w173:T11)
                n172 = call "日志存储 (子VI).vi"("data in"=w173) -> ()  [unwired: 11 in]
              }
              frame #1 {
                n173 = call "Force Quit LabVIEW.vi"() -> ()  [unwired: 10 in, 2 out]
              }
              frame #2 {
                n174 = Quit LabVIEW(quit? (T)=TRUE ("退出？(T)")) -> ()
              }
            }
          }
        }
        n175 = event-data("Discard?"=w163) -> ()  [unwired: 1 in, 1 out]
      }
      event "站点名称", "站点设备", "IP", "PORT", "MN", "PW", "VISA resource name", "baud rate", "系统编码选择框", "每周自动重发", "重发日期", "重发时间", "暂停上传": Value Change {
        n176 = event-data() -> ("CtlRef"=w177:refnum<vi>)  [unwired: 1 in, 5 out]
        n177 = flat-sequence {
          tunnel: w177 -> [w179]
          tunnel: [w178] -> w176
          tunnel: w176 -> [w193]
          frame #0 {
            n178 = property class="Ctl"(reference=w179) -> ("Caption.Text"=w178:string)  [unwired: 1 in, 2 out]
            n179 = global write "断电保存全局.vi" "IP"("IP") -> ()
            n180 = global write "断电保存全局.vi" "PORT"("PORT") -> ()
            n181 = global write "断电保存全局.vi" "MN"("MN") -> ()
            n182 = global write "断电保存全局.vi" "站点设备"("站点设备") -> ()
            n183 = global write "断电保存全局.vi" "PW"("PW") -> ()
            n184 = global write "断电保存全局.vi" "重发时间"("重发时间") -> ()
            n185 = global write "断电保存全局.vi" "暂停上传"("暂停上传") -> ()
            n186 = global write "断电保存全局.vi" "重发日期"("重发日期") -> ()
            n187 = global write "断电保存全局.vi" "站点名称"("站点名称") -> ()
            n188 = global write "断电保存全局.vi" "baud rate"("baud rate") -> ()
            n189 = global write "断电保存全局.vi" "系统编码选择框"("系统编码选择框") -> ()
            n190 = global write "断电保存全局.vi" "每周自动重发"("每周自动重发") -> ()
            n191 = global write "断电保存全局.vi" "VISA resource name"("VISA resource name") -> ()
          }
          frame #1 {
            n192 = case shown="\"IP\", \"PORT\"" w193 {
              selector: w193 -> [_ w194]
              frame "假", Default {
              }
              frame "IP", "PORT" {
                n193 = call "通信状态入队列.vi"("发送报文"=w194, "枚举"=enum16{"打开连接", "发送数据", "读取数据", "数据处理", "关闭连接"}."关闭连接") -> ()  [unwired: 9 in, 1 out]
              }
            }
            n194 = call "配置文件断电保存(子VI).vi"() -> ()  [unwired: 12 in]
          }
        }
      }
      event "数据发送通道", "数据发送协议", "数据组合发送", "2011发送", "自动更新": Value Change {
        n195 = event-data() -> ("CtlRef"=w199:refnum<vi>, "OldVal"=w197:variant, "NewVal"=w196:variant)  [unwired: 1 in, 3 out]
        n196 = property class="Ctl"(reference=w199) -> ("Label.Text"=w198:string)  [unwired: 1 in, 2 out]
        n197 = case shown="\"自动更新\"" w198 {
          tunnel: w197 -> [_ w203 w226 w235 w261 w285 w308 w329]
          tunnel: w196 -> [_ w200 w223 w232 w259 w282 w305 w328]
          frame "假", Default {
          }
          frame "数据发送通道" {
            n198 = Variant To Data(type=enum16{"TCP", "VISA"}."TCP" ("数据发送通道"), Variant=w200) -> (data=w201:enum16{"TCP", "VISA"})  [unwired: 1 in, 1 out]
            n199 = global write "断电保存全局.vi" "数据发送通道"(w201) -> ()
            n200 = Two Button Dialog(message="TCP通过网络发送数据，VISA通过串口发送数据，确定更改数据发送通道吗？" ("消息")) -> (T button?=w204:bool)  [unwired: 2 in]
            n201 = case shown="假" w204 {
              tunnel: w203 -> [w207 _]
              frame False {
                n202 = Variant To Data(type=enum16{"TCP", "VISA"}."TCP" ("数据发送通道"), Variant=w207) -> (data=w206:enum16{"TCP", "VISA"})  [unwired: 1 in, 1 out]
                n203 = global write "断电保存全局.vi" "数据发送通道"(w206) -> ()
              }
              frame True {
                n204 = flat-sequence {
                  frame #0 {
                  }
                  frame #1 {
                    n205 = call <vilib>:"Application Directory.vi"() -> ("Application Directory"=w209:path)
                    n206 = Build Path(base path=w209, name or relative path="data\\sys.ini" ("名称或相对路径")) -> (appended path=w211:path)
                    n207 = call <vilib>:"Open Config Data.vi"("configuration file path"=w211) -> ("error out"=w215:errorcluster, "refnum"=w212:T13)  [unwired: 8 in, 1 out]
                    n208 = vi-ref "断电保存全局.vi"() -> (w213:refnum<vi>)
                    n209 = call <userlib>:"Write Panel to INI__ogtk.vi"("error in (no error)"=w215, "VI ref"=w213, "refnum"=w212) -> ("error out"=w216:errorcluster, "refnum out"=w214:T13)  [unwired: 7 in]
                    n210 = call <vilib>:"Close Config Data.vi"("error in (no error)"=w216, "refnum"=w214) -> ("error out"=w221:errorcluster, "file path"=w222:path)  [unwired: 8 in]
                    n211 = Open/Create/Replace File(file path (use dialog)=w222, error in=w221) -> (refnum out=w218:refnum<file>, error out=w217:errorcluster)  [unwired: 4 in, 1 out]
                    n212 = Flush File(refnum=w218, error in=w217) -> (refnum out=w219:refnum<file>, error out=w220:errorcluster)
                    n213 = Close File(refnum=w219, error in=w220) -> ()  [unwired: 2 out]
                  }
                }
              }
            }
          }
          frame "数据发送协议" {
            n214 = Variant To Data(type=enum16{"2005-212协议", "2017-212协议"}."2017-212协议" ("数据"), Variant=w223) -> (data=w224:enum16{"2005-212协议", "2017-212协议"})  [unwired: 1 in, 1 out]
            n215 = global write "断电保存全局.vi" "数据发送协议"(w224) -> ()
            n216 = Two Button Dialog(message="2005对应旧版通信协议，2017对应最新版协议，对应协议因子编码会不同，\n更改可能导致数据不能被平台识别，确定更改数据发送协议吗？" ("消息")) -> (T button?=w227:bool)  [unwired: 2 in]
            n217 = case shown="真" w227 {
              tunnel: w226 -> [w231 _]
              frame False {
                n218 = Variant To Data(type=enum16{"2005-212协议", "2017-212协议"}."2017-212协议" ("数据"), Variant=w231) -> (data=w229:enum16{"2005-212协议", "2017-212协议"})  [unwired: 1 in, 1 out]
                n219 = global write "断电保存全局.vi" "数据发送协议"(w229) -> ()
              }
              frame True {
                n220 = call "配置文件断电保存(子VI).vi"() -> ()  [unwired: 12 in]
              }
            }
          }
          frame "数据组合发送" {
            n221 = Variant To Data(type=FALSE, Variant=w232) -> (data=w233:bool)  [unwired: 1 in, 1 out]
            n222 = global write "断电保存全局.vi" "数据组合发送"(w233) -> ()
            n223 = Two Button Dialog(message="勾选数据组合发送功能表示所有参数打包整点同时上传、则只能整点发送延时较高，\n不勾选则表示单参数分别上传、则实时性较好，确定更改数据组合发送功能吗？" ("消息")) -> (T button?=w236:bool)  [unwired: 2 in]
            n224 = case shown="真" w236 {
              tunnel: w235 -> [w239 _]
              frame False {
                n225 = Variant To Data(type=FALSE, Variant=w239) -> (data=w238:bool)  [unwired: 1 in, 1 out]
                n226 = global write "断电保存全局.vi" "数据组合发送"(w238) -> ()
              }
              frame True {
                n227 = flat-sequence {
                  frame #0 {
                  }
                  frame #1 {
                    n228 = call <vilib>:"Application Directory.vi"() -> ("Application Directory"=w241:path)
                    n229 = Build Path(base path=w241, name or relative path="data\\sys.ini" ("名称或相对路径")) -> (appended path=w243:path)
                    n230 = call <vilib>:"Open Config Data.vi"("configuration file path"=w243) -> ("error out"=w247:errorcluster, "refnum"=w244:T13)  [unwired: 8 in, 1 out]
                    n231 = vi-ref "断电保存全局.vi"() -> (w245:refnum<vi>)
                    n232 = call <userlib>:"Write Panel to INI__ogtk.vi"("error in (no error)"=w247, "VI ref"=w245, "refnum"=w244) -> ("error out"=w248:errorcluster, "refnum out"=w246:T13)  [unwired: 7 in]
                    n233 = call <vilib>:"Close Config Data.vi"("error in (no error)"=w248, "refnum"=w246) -> ("error out"=w253:errorcluster, "file path"=w254:path)  [unwired: 8 in]
                    n234 = Open/Create/Replace File(file path (use dialog)=w254, error in=w253) -> (refnum out=w250:refnum<file>, error out=w249:errorcluster)  [unwired: 4 in, 1 out]
                    n235 = Flush File(refnum=w250, error in=w249) -> (refnum out=w251:refnum<file>, error out=w252:errorcluster)
                    n236 = Close File(refnum=w251, error in=w252) -> ()  [unwired: 2 out]
                  }
                }
              }
            }
          }
          frame "自动更新" {
            n237 = Variant To Data(type=FALSE, Variant=w259) -> (data=w257:bool)  [unwired: 1 in, 1 out]
            n238 = global write "断电保存全局.vi" "自动更新"(w257) -> ()
            n239 = case shown="假" w257 {
              tunnel: ["关闭" "启用"] -> w256
              frame False {
              }
              frame True {
              }
            }
            n240 = Format Into String(format string="每周一0-6点间自动更新，确认%s？" ("消息"), w256) -> (resulting string=w255:string)  [unwired: 2 in, 1 out]
            n241 = Two Button Dialog(message=w255) -> (T button?=w262:bool)  [unwired: 2 in]
            n242 = case shown="真" w262 {
              tunnel: w261 -> [w266 _]
              frame False {
                n243 = Variant To Data(type=FALSE, Variant=w266) -> (data=w265:bool)  [unwired: 1 in, 1 out]
                n244 = global write "断电保存全局.vi" "自动更新"(w265) -> ()
              }
              frame True {
                n245 = flat-sequence {
                  frame #0 {
                  }
                  frame #1 {
                    n246 = call <vilib>:"Application Directory.vi"() -> ("Application Directory"=w268:path)
                    n247 = Build Path(base path=w268, name or relative path="data\\sys.ini" ("名称或相对路径")) -> (appended path=w270:path)
                    n248 = call <vilib>:"Open Config Data.vi"("configuration file path"=w270) -> ("error out"=w274:errorcluster, "refnum"=w271:T13)  [unwired: 8 in, 1 out]
                    n249 = vi-ref "断电保存全局.vi"() -> (w272:refnum<vi>)
                    n250 = call <userlib>:"Write Panel to INI__ogtk.vi"("error in (no error)"=w274, "VI ref"=w272, "refnum"=w271) -> ("error out"=w275:errorcluster, "refnum out"=w273:T13)  [unwired: 7 in]
                    n251 = call <vilib>:"Close Config Data.vi"("error in (no error)"=w275, "refnum"=w273) -> ("error out"=w280:errorcluster, "file path"=w281:path)  [unwired: 8 in]
                    n252 = Open/Create/Replace File(file path (use dialog)=w281, error in=w280) -> (refnum out=w277:refnum<file>, error out=w276:errorcluster)  [unwired: 4 in, 1 out]
                    n253 = Flush File(refnum=w277, error in=w276) -> (refnum out=w278:refnum<file>, error out=w279:errorcluster)
                    n254 = Close File(refnum=w278, error in=w279) -> ()  [unwired: 2 out]
                  }
                }
              }
            }
          }
          frame "2011发送" {
            n255 = Variant To Data(type=FALSE, Variant=w282) -> (data=w283:bool)  [unwired: 1 in, 1 out]
            n256 = global write "断电保存全局.vi" "2011发送"(w283) -> ()
            n257 = Two Button Dialog(message="2011表示实时数据上传，一般情况需要勾选，确定更改2011实时数据发送功能吗？" ("消息")) -> (T button?=w286:bool)  [unwired: 2 in]
            n258 = case shown="真" w286 {
              tunnel: w285 -> [w289 _]
              frame False {
                n259 = Variant To Data(type=FALSE, Variant=w289) -> (data=w288:bool)  [unwired: 1 in, 1 out]
                n260 = global write "断电保存全局.vi" "2011发送"(w288) -> ()
              }
              frame True {
                n261 = flat-sequence {
                  frame #0 {
                  }
                  frame #1 {
                    n262 = call <vilib>:"Application Directory.vi"() -> ("Application Directory"=w291:path)
                    n263 = Build Path(base path=w291, name or relative path="data\\sys.ini" ("名称或相对路径")) -> (appended path=w293:path)
                    n264 = call <vilib>:"Open Config Data.vi"("configuration file path"=w293) -> ("error out"=w297:errorcluster, "refnum"=w294:T13)  [unwired: 8 in, 1 out]
                    n265 = vi-ref "断电保存全局.vi"() -> (w295:refnum<vi>)
                    n266 = call <userlib>:"Write Panel to INI__ogtk.vi"("error in (no error)"=w297, "VI ref"=w295, "refnum"=w294) -> ("error out"=w298:errorcluster, "refnum out"=w296:T13)  [unwired: 7 in]
                    n267 = call <vilib>:"Close Config Data.vi"("error in (no error)"=w298, "refnum"=w296) -> ("error out"=w303:errorcluster, "file path"=w304:path)  [unwired: 8 in]
                    n268 = Open/Create/Replace File(file path (use dialog)=w304, error in=w303) -> (refnum out=w300:refnum<file>, error out=w299:errorcluster)  [unwired: 4 in, 1 out]
                    n269 = Flush File(refnum=w300, error in=w299) -> (refnum out=w301:refnum<file>, error out=w302:errorcluster)
                    n270 = Close File(refnum=w301, error in=w302) -> ()  [unwired: 2 out]
                  }
                }
              }
            }
          }
          frame "日志、参数发送" {
            n271 = Variant To Data(type=FALSE, Variant=w305) -> (data=w306:bool)  [unwired: 1 in, 1 out]
            n272 = global write "断电保存全局.vi" "日志、参数发送"(w306) -> ()
            n273 = Two Button Dialog(message="选择是否需要仪器日志、状态和告警信息上传，一般情况需要勾选，确定更改日志、参数发送功能吗？" ("消息")) -> (T button?=w309:bool)  [unwired: 2 in]
            n274 = case shown="假" w309 {
              tunnel: w308 -> [w312 _]
              frame False {
                n275 = Variant To Data(type=FALSE, Variant=w312) -> (data=w311:bool)  [unwired: 1 in, 1 out]
                n276 = global write "断电保存全局.vi" "日志、参数发送"(w311) -> ()
              }
              frame True {
                n277 = flat-sequence {
                  frame #0 {
                  }
                  frame #1 {
                    n278 = call <vilib>:"Application Directory.vi"() -> ("Application Directory"=w314:path)
                    n279 = Build Path(base path=w314, name or relative path="data\\sys.ini" ("名称或相对路径")) -> (appended path=w316:path)
                    n280 = call <vilib>:"Open Config Data.vi"("configuration file path"=w316) -> ("error out"=w320:errorcluster, "refnum"=w317:T13)  [unwired: 8 in, 1 out]
                    n281 = vi-ref "断电保存全局.vi"() -> (w318:refnum<vi>)
                    n282 = call <userlib>:"Write Panel to INI__ogtk.vi"("error in (no error)"=w320, "VI ref"=w318, "refnum"=w317) -> ("error out"=w321:errorcluster, "refnum out"=w319:T13)  [unwired: 7 in]
                    n283 = call <vilib>:"Close Config Data.vi"("error in (no error)"=w321, "refnum"=w319) -> ("error out"=w326:errorcluster, "file path"=w327:path)  [unwired: 8 in]
                    n284 = Open/Create/Replace File(file path (use dialog)=w327, error in=w326) -> (refnum out=w323:refnum<file>, error out=w322:errorcluster)  [unwired: 4 in, 1 out]
                    n285 = Flush File(refnum=w323, error in=w322) -> (refnum out=w324:refnum<file>, error out=w325:errorcluster)
                    n286 = Close File(refnum=w324, error in=w325) -> ()  [unwired: 2 out]
                  }
                }
              }
            }
          }
          frame "判断数据反馈" {
            n287 = Two Button Dialog(message="判断数据反馈是针对平台能有反馈的情况，\n1.严格判断反馈-收不到反馈一直重发\n2.非严格判断-重发5次后跳过该数据\n3.不判断反馈针对平台没有反馈的情况\n确定更改判断数据反馈功能吗？" ("消息")) -> (T button?=w330:bool)  [unwired: 2 in]
            n288 = case shown="假" w330 {
              tunnel: w329 -> [_ _]
              tunnel: w328 -> [w333 w335]
              frame False {
                n289 = Variant To Data(type=enum16{"非严格判断", "严格判断", "不判断"}."非严格判断" ("判断数据反馈"), Variant=w333) -> (data=w332:enum16{"非严格判断", "严格判断", "不判断"})  [unwired: 1 in, 1 out]
                n290 = local write "判断数据反馈"(w332) -> ()
              }
              frame True {
                n291 = flat-sequence {
                  tunnel: w335 -> [w336]
                  frame #0 {
                    n292 = Variant To Data(type=enum16{"非严格判断", "严格判断", "不判断"}."非严格判断" ("判断数据反馈"), Variant=w336) -> (data=w338:enum16{"非严格判断", "严格判断", "不判断"})  [unwired: 1 in, 1 out]
                    n293 = global write "断电保存全局.vi" "判断数据反馈"(w338) -> ()
                  }
                  frame #1 {
                    n294 = call <vilib>:"Application Directory.vi"() -> ("Application Directory"=w339:path)
                    n295 = Build Path(base path=w339, name or relative path="data\\sys.ini" ("名称或相对路径")) -> (appended path=w341:path)
                    n296 = call <vilib>:"Open Config Data.vi"("configuration file path"=w341) -> ("error out"=w345:errorcluster, "refnum"=w342:T13)  [unwired: 8 in, 1 out]
                    n297 = vi-ref "断电保存全局.vi"() -> (w343:refnum<vi>)
                    n298 = call <userlib>:"Write Panel to INI__ogtk.vi"("error in (no error)"=w345, "VI ref"=w343, "refnum"=w342) -> ("error out"=w346:errorcluster, "refnum out"=w344:T13)  [unwired: 7 in]
                    n299 = call <vilib>:"Close Config Data.vi"("error in (no error)"=w346, "refnum"=w344) -> ("error out"=w351:errorcluster, "file path"=w352:path)  [unwired: 8 in]
                    n300 = Open/Create/Replace File(file path (use dialog)=w352, error in=w351) -> (refnum out=w348:refnum<file>, error out=w347:errorcluster)  [unwired: 4 in, 1 out]
                    n301 = Flush File(refnum=w348, error in=w347) -> (refnum out=w349:refnum<file>, error out=w350:errorcluster)
                    n302 = Close File(refnum=w349, error in=w350) -> ()  [unwired: 2 out]
                  }
                }
              }
            }
          }
        }
      }
      event "确定": Value Change {
        n303 = event-data() -> ()  [unwired: 1 in, 6 out]
        n304 = call "通信状态入队列.vi"("枚举"=enum16{"打开连接", "发送数据", "读取数据", "数据处理", "关闭连接"}."关闭连接") -> ()  [unwired: 10 in, 1 out]
      }
      event "配置表": Value Change {
        n305 = event-data() -> ()  [unwired: 1 in, 6 out]
        n306 = call "参数配置表.vi"() -> ()  [unwired: 12 in]
      }
      event "参数配置": Value Change {
        n307 = event-data() -> ()  [unwired: 1 in, 6 out]
        n308 = property on="窗格" class="Pane"("Origin"=T7 {"Horizontal"=0, "Vertical"=1000} ("原点")) -> ()  [unwired: 2 in, 2 out]
        n309 = call <vilib>:"Application Directory.vi"() -> ("Application Directory"=w355:path)
        n310 = call "查询启动项.vi"("启动文件路径"=w355) -> ("包含启动项"=w354:bool)  [unwired: 9 in, 1 out]
        n311 = local write "开机启动"(w354) -> ()
      }
      event "返回": Value Change {
        n312 = event-data() -> ()  [unwired: 1 in, 6 out]
        n313 = property on="窗格" class="Pane"("Origin"=T7 {"Horizontal"=0, "Vertical"=0} ("原点")) -> ()  [unwired: 2 in, 2 out]
      }
      event "数据补传": Value Change {
        n314 = event-data() -> ()  [unwired: 1 in, 6 out]
        n315 = global read "全局1.vi" "数据发送起始时间"() -> (w358:timestamp)
        n316 = call "数据补传对话框.vi"("起始时间"=w358) -> ("结束时间输出"=w359:timestamp, "起始时间输出"=w360:timestamp, "输出"=w361:bool)  [unwired: 8 in]
        n317 = case shown="真" w361 {
          tunnel: w360 -> [_ w363]
          tunnel: w359 -> [_ w368]
          frame False {
          }
          frame True {
            w362 = TRUE ("数据重发")
            n318 = global write "全局1.vi" "数据发送起始时间"(w363) -> ()
            n319 = global write "断电保存全局.vi" "数据重发结束时间"(w368) -> ()
            n320 = global write "断电保存全局.vi" "数据重发"(w362) -> ()
            n321 = global write "断电保存全局.vi" "日志信息重发"(w362) -> ()
            n322 = global write "断电保存全局.vi" "剖面数据重发"(w362) -> ()
            n323 = global read "断电保存全局.vi" "数据组合发送"() -> (w376:bool)
            n324 = Format Date/Time String(time format string (%c)="%Y/%m/%d %H:%M:%S" ("时间格式字符串(%c)"), seconds (now)=w363) -> (date/time string=w364:string)  [unwired: 1 in]
            n325 = case shown="假" w376 {
              tunnel: w364 -> [w377 _]
              frame False {
                n326 = global write "全局 时间2.vi" "标样核查索引起始时间"(w377) -> ()
                n327 = global write "全局 时间2.vi" "加标回收索引起始时间"(w377) -> ()
                n328 = global write "全局 时间2.vi" "跨度核查索引起始时间"(w377) -> ()
                n329 = global write "全局 时间2.vi" "3092日志索引起始时间"(w377) -> ()
                n330 = global write "全局 时间2.vi" "零点核查索引起始时间"(w377) -> ()
                n331 = Initialize Array(w377, 9 ("维数大小")) -> (w389:string[])
                n332 = Initialize Array(w377, 6 ("维数大小")) -> (w381:string[])
                n333 = Initialize Array(w377, 7 ("维数大小")) -> (w380:string[])
                n334 = Initialize Array(w377, 16 ("维数大小")) -> (w384:string[])
                n335 = Array To Cluster(array=w380) -> (cluster=w379:T14)
                n336 = Array To Cluster(array=w389) -> (cluster=w388:T15)
                n337 = Array To Cluster(array=w381) -> (cluster=w382:T16)
                n338 = global write "全局 时间2.vi" "跨度核查索引"(w388) -> ()
                n339 = global write "全局 时间2.vi" "零点核查索引"(w388) -> ()
                n340 = global write "全局 时间2.vi" "平行样索引"(w382) -> ()
                n341 = global write "全局 时间2.vi" "加标回收索引"(w382) -> ()
                n342 = global write "全局 时间2.vi" "仪器日志索引"(w379) -> ()
                n343 = Array To Cluster(array=w384) -> (cluster=w385:T17)
                n344 = global write "全局 时间2.vi" "标样核查索引"(w385) -> ()
                n345 = global write "全局 时间2.vi" "集成干预索引"(w385) -> ()
              }
              frame True {
              }
            }
            n346 = global write "全局 水样时间.vi" "剖面多参数数据时间"(w364) -> ()
            n347 = global write "全局 水样时间.vi" "剖面数据时间"(w364) -> ()
            n348 = global write "断电保存全局.vi" "数据重发时间戳"(w364) -> ()
            n349 = Initialize Array(w364, 14 ("维数大小")) -> (w369:string[])
            n350 = Initialize Array(w364, 35 ("维数大小")) -> (w373:string[])
            n351 = Initialize Array(w364, 7 ("维数大小")) -> (w367:string[])
            n352 = Array To Cluster(array=w367) -> (cluster=w366:T14)
            n353 = global write "全局 时间2.vi" "仪器日志索引"(w366) -> ()
            n354 = Array To Cluster(array=w369) -> (cluster=w370:T18)
            n355 = Array To Cluster(array=w373) -> (cluster=w372:T19)
            n356 = global write "全局 时间2.vi" "仪器参数索引"(w370) -> ()
            n357 = global write "全局 水样时间.vi" "水样数据索引"(w372) -> ()
          }
        }
      }
      event "开机启动": Value Change {
        n358 = event-data() -> ("CtlRef"=w391:refnum<vi>, "OldVal"=w390:bool, "NewVal"=w392:bool)  [unwired: 1 in, 3 out]
        n359 = case shown="真" w392 {
          tunnel: w391 -> [w394 w407]
          tunnel: w390 -> [w393 w406]
          frame False {
            n360 = Two Button Dialog(message="是否删除开机启动？" ("消息"), 1:"否" ("F按钮名称（“取消”）"), 2:"是" ("T按钮名称（“确定”）")) -> (T button?=w395:bool)
            n361 = case shown="假" w395 {
              tunnel: w394 -> [w400 _]
              tunnel: w393 -> [w399 _]
              frame False {
                n362 = property class="Bool (严格)"(reference=w400, "Value"=w399) -> ()  [unwired: 1 in, 2 out]
              }
              frame True {
                n363 = call <vilib>:"Application Directory.vi"() -> ("Application Directory"=w402:path)
                n364 = call "删除启动项.vi"("启动文件路径"=w402) -> ("删除标记"=w401:bool)  [unwired: 9 in, 1 out]
                n365 = case shown="假" w401 {
                  tunnel: ["删除开机启动失败" ("T按钮名称（“确定”）") "删除开机启动成功" ("T按钮名称（“确定”）")] -> w403
                  frame False {
                  }
                  frame True {
                  }
                }
                n366 = One Button Dialog(message=w403) -> ()  [unwired: 1 in, 1 out]
              }
            }
          }
          frame True {
            n367 = Two Button Dialog(message="是否添加开机启动？" ("消息"), 1:"否" ("F按钮名称（“取消”）"), 2:"是" ("T按钮名称（“确定”）")) -> (T button?=w408:bool)
            n368 = case shown="真" w408 {
              tunnel: w407 -> [w413 _]
              tunnel: w406 -> [w412 _]
              frame False {
                n369 = property class="Bool (严格)"(reference=w413, "Value"=w412) -> ()  [unwired: 1 in, 2 out]
              }
              frame True {
                n370 = call <vilib>:"Application Directory.vi"() -> ("Application Directory"=w416:path)
                n371 = call "添加启动项.vi"("启动文件路径"=w416) -> ("添加成功标记"=w415:bool)  [unwired: 9 in, 1 out]
                n372 = case shown="真" w415 {
                  tunnel: ["添加开机启动失败" ("T按钮名称（“确定”）") "添加开机启动成功" ("T按钮名称（“确定”）")] -> w414
                  frame False {
                  }
                  frame True {
                  }
                }
                n373 = One Button Dialog(message=w414) -> ()  [unwired: 1 in, 1 out]
              }
            }
          }
        }
      }
      event "更新": Value Change {
        n374 = event-data() -> ()  [unwired: 1 in, 6 out]
        n375 = call "自定义双按钮对话框.vi"("消息"="选择是否从服务器获取最新版本信息？") -> ("正式版/测试版输出"=w419:bool, "输出"=w420:bool)  [unwired: 9 in]
        n376 = case shown="真" w420 {
          tunnel: w419 -> [_ w422]
          frame False {
          }
          frame True {
            w431 = T20 2 items=["两端", "字符串首端", "字符串末端"] ("location (both)")
            w427 = "/" ("分隔符(Tab)")
            # "获取最新版本"
            n377 = local read "updateconfiguration"() -> (w439:T1)
            n378 = Unbundle By Name(w439) -> ("主机"=w438:string, "用户"=w428:string, "密码"=w437:string, "远程路径"=w435:string)
            n379 = Spreadsheet String To Array(delimiter (Tab)="\\" ("分隔符(Tab)"), format string="" ("格式字符串"), spreadsheet string=w435, array type (2D Dbl)=string[] []) -> (array=w424:string[])
            n380 = case shown="真" w422 {
              tunnel: w424 -> [w442 w444]
              tunnel: [w442 w443] -> w423
              frame False {
                # "正式版"
              }
              frame True {
                # "测试版"
                n381 = Array Size(array=w444) -> (size(s)=w445:i32)
                n382 = Subtract(x=w445, y=2) -> (x-y=w447:i32)
                n383 = Index Array(array=w444, index=w447) -> (element=w448:string)
                n384 = Concatenate Strings(w448, "beta" ("字符串")) -> (w450:string)
                n385 = Replace Array Subset(array=w444, new element=w450, index=w447) -> (w443:string[])
              }
            }
            n386 = Array To Spreadsheet String(delimiter (Tab)=w427, array=w423, 3:"%s" ("格式字符串")) -> (spreadsheet string=w426:string)
            n387 = Concatenate Strings(w427, w426) -> (w425:string)
            n388 = call <vilib>:"Trim Whitespace.vi"("string"=w425, "location (both)"=w431) -> ("trimmed string"=w430:string)
            n389 = Bundle By Name(cluster=T12 {"host"="27.154.58.30", "port"=8020, "user"="std", "password"="std23506", "远端地址"="/微站/室外总磷总氮高压过滤无主板新电路板/一体化微型水质监测站.exe"} ("服务器信息"), "host"=w438, "port"=u16 8020, "user"=w428, "password"=w437, "远端地址"=w430) -> (w440:T12)
            n390 = call "Update.vi"("测试版？"=w422, "服务器信息"=w440) -> ()  [unwired: 10 in]
          }
        }
      }
      event "updateconfiguration": Value Change {
        n391 = event-data() -> ("NewVal"=w458:T1)  [unwired: 1 in, 5 out]
        n392 = call <vilib>:"Application Directory.vi"() -> ("Application Directory"=w462:path)
        n393 = Build Path(base path=w462, name or relative path="update\\data\\set.ini" ("名称或相对路径")) -> (appended path=w460:path)
        n394 = Build Array("主机" ("section"), "用户" ("section"), "密码" ("key"), "远程路径" ("key"), "下载文件名" ("key"), "软件版本" ("key")) -> (w451:string[])
        n395 = call "配置文件write.vi"("updateconfiguration"=w458, "configuration file path"=w460, "键数组"=w451, "段"="应用程序交互" ("section")) -> ("error out"=w459:errorcluster)  [unwired: 7 in]
        n396 = call <vilib>:"Clear Errors.vi"("error in (no error)"=w459) -> ()  [unwired: 5 in, 2 out]
      }
      event "IP", "PORT": Mouse Down {
        n397 = event-data() -> ("CtlRef"=w472:refnum<vi>)  [unwired: 1 in, 7 out]
        n398 = property class="Str"(reference=w472) -> (reference out=w470:refnum<vi>, "Value"=w471:string)  [unwired: 1 in, 1 out]
        n399 = call "IP键盘.vi"("OldNumber"=w471) -> ("NewNumber"=w467:string)
        n400 = String Length(string=w467) -> (length=w469:i32)
        n401 = Less Or Equal?(x=w469, y=15) -> (x <= y?=w466:bool)
        n402 = case shown="假" w466 {
          tunnel: w470 -> [w473 w477]
          tunnel: w467 -> [_ w476]
          tunnel: [w473 w477] -> w465
          tunnel: ["127.0.0.1" w476] -> w464
          frame False {
            n403 = One Button Dialog(message="超过ipv4最大长度限制,请重新输入!" ("消息")) -> ()  [unwired: 1 in, 1 out]
          }
          frame True {
          }
        }
        n404 = property class="Str"(reference=w465, "Val(Sgnl)"=w464) -> ()  [unwired: 1 in, 2 out]
      }
    }
  }
  n405 = while {
    shift-right: [w482] -> _
    shift-left: "数  据  采  集  传  输  系  统" ("标题显示") -> [w483]
    stop <- FALSE stop-if-true
    n406 = global read "断电保存全局.vi" "数据重发"() -> (w480:bool)
    n407 = global read "断电保存全局.vi" "剖面数据重发"() -> (w478:bool)
    n408 = global read "断电保存全局.vi" "日志信息重发"() -> (w479:bool)
    n409 = call "字符串移位显示.vi"("字符框大小"=72, "字符串输入"=w483) -> ("移位后字符串"=w482:string)  [unwired: 8 in, 1 out]
    "标题显示" <- w482
    n410 = Wait (ms)(milliseconds to wait=u32 1000 ("等待时间（毫秒）")) -> ()  [unwired: 1 out]
    n411 = property on="数据补发" class="Bool (严格)"("Visible"=w480, "Value"=w480) -> ()  [unwired: 2 in, 2 out]
    n412 = property on="剖面数据补发" class="Bool (严格)"("Visible"=w478, "Value"=w478) -> ()  [unwired: 2 in, 2 out]
    n413 = property on="日志信息补发" class="Bool (严格)"("Visible"=w479, "Value"=w479) -> ()  [unwired: 2 in, 2 out]
  }
